vi "Init GUIs.vi"(0 "Windows in":T1, 1 "JSON":refnum<class "ConfigJSON.lvclass">, 2 "SVW":refnum<class "SharedVariableWrapper.lvclass">, 11 "error in":errorcluster) -> (4 "Windows out":T1, 15 "error out":errorcluster)   [LabVIEW 2019]
uses:
  TypeDef/Windows.ctl
  GUI Sensor Lib/GUI Sensor Lib.lvclass
  D:/GIT H4000/H4000/src/GUI_class/GUI.lvclass
  GUI Alarm Setting/GUI Alarm Setting.lvclass
  GUI Data Viewer_class/GUI Data Viewer.lvclass
  GUI Test Channels_class/GUI Test Channels.lvclass
  GUI Setting_class/GUI Setting.lvclass
  GUI Test HIPRESS_class/GUI Test HIPRESS.lvclass
  GUI NV class/GUI NV.lvclass
  GUI Work Windows_class/GUI Work Windows.lvclass
  PumpMotorGroup_class/GUI PumpMotorGroup.lvclass
  SV_Wrap/SharedVariableWrapper.lvclass
  ConfigJSON_class/ConfigJSON.lvclass
  D:/GIT H4000/H4000/src/ConfigInterface_class/ConfigInterface.lvclass
  GUI_class/GUI.lvclass/GUI.ctl
  GUI_class/GUI.lvclass
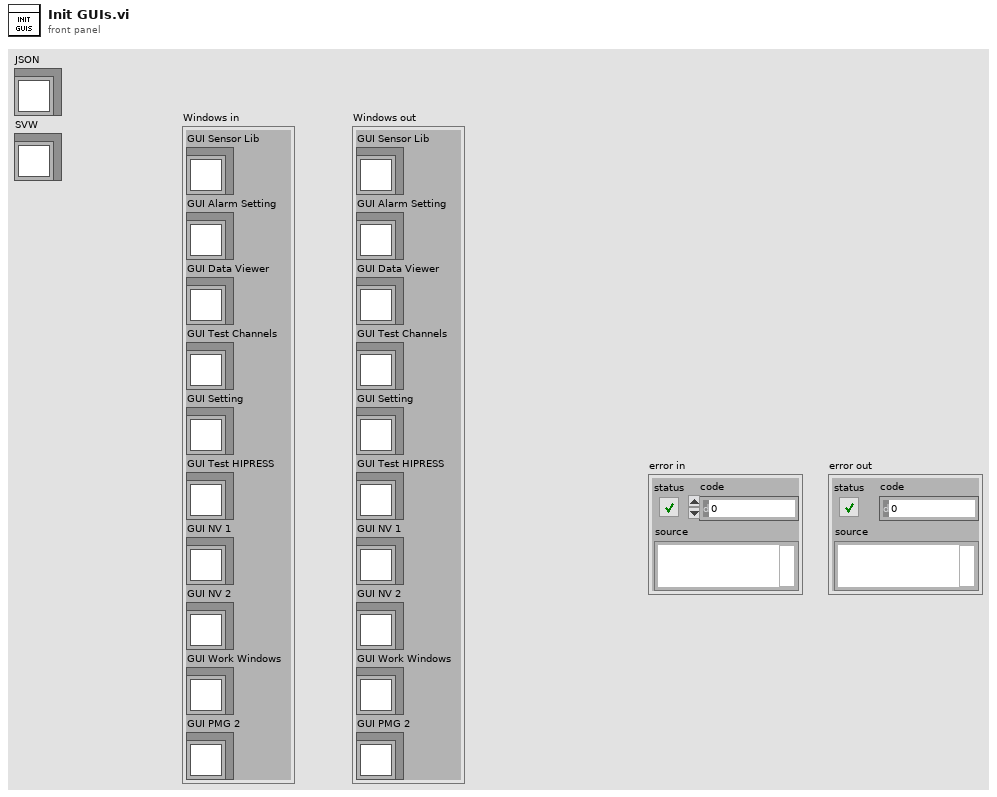
[diagram p1: front panel]
types:
  T1 = typedef "Windows.ctl" = cluster{"GUI Sensor Lib":refnum<class "GUI Sensor Lib.lvclass">, "GUI Alarm Setting":refnum<class "GUI Alarm Setting.lvclass">, "GUI Data Viewer":refnum<class "GUI Data Viewer.lvclass">, "GUI Test Channels":refnum<class "GUI Test Channels.lvclass">, "GUI Setting":refnum<class "GUI Setting.lvclass">, "GUI Test HIPRESS":refnum<class "GUI Test HIPRESS.lvclass">, "GUI NV 1":refnum<class "GUI NV.lvclass">, "GUI NV 2":refnum<class "GUI NV.lvclass">, "GUI Work Windows":refnum<class "GUI Work Windows.lvclass">, "GUI PMG 2":refnum<class "GUI PumpMotorGroup.lvclass">}
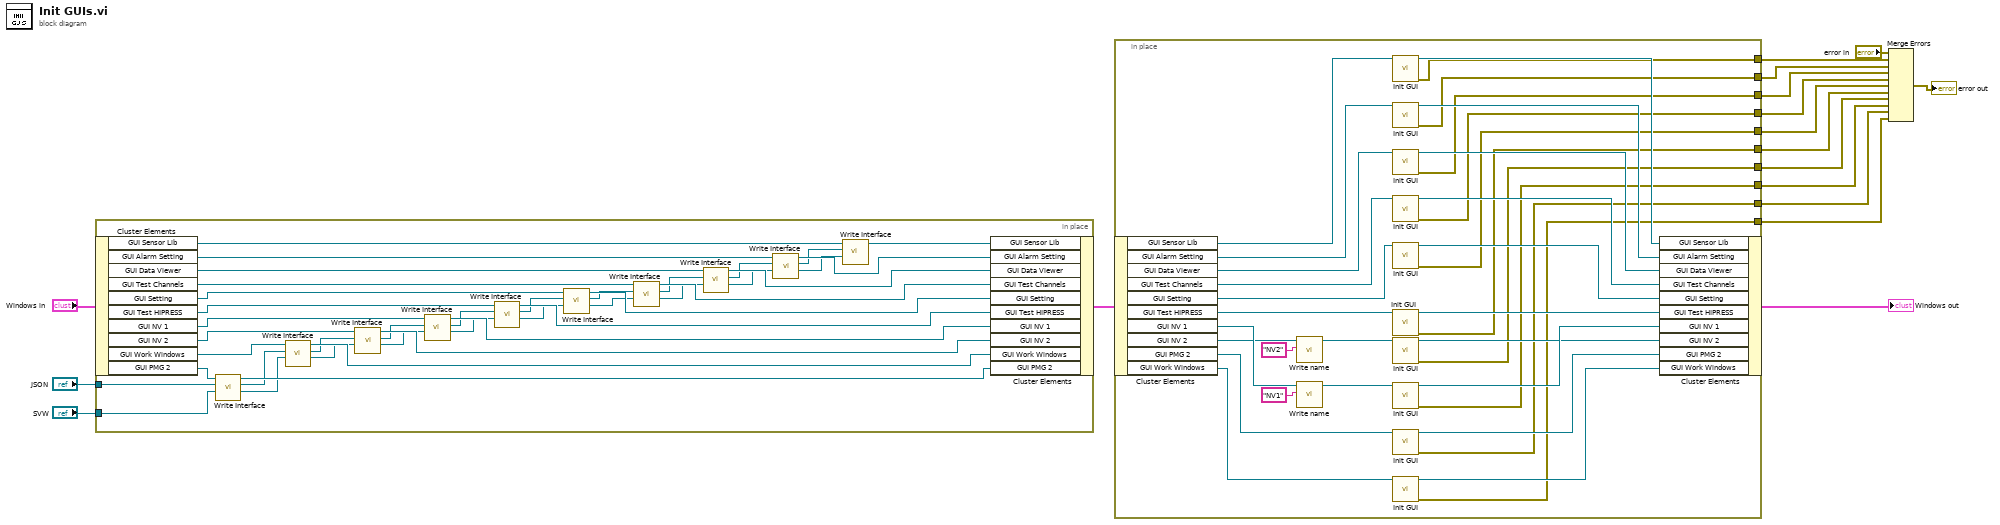
[diagram p0: block diagram]
diagram:
  n1 = in-place {
    in-place-border: "JSON" -> [w37]
    in-place-border: "SVW" -> [w36]
    n2 = in-place-cluster #1("Windows in") -> ("GUI Sensor Lib"=w57:refnum<class "GUI Sensor Lib.lvclass">, "GUI Alarm Setting"=w55:refnum<class "GUI Alarm Setting.lvclass">, "GUI Data Viewer"=w54:refnum<class "GUI Data Viewer.lvclass">, "GUI Test Channels"=w53:refnum<class "GUI Test Channels.lvclass">, "GUI Setting"=w52:refnum<class "GUI Setting.lvclass">, "GUI Test HIPRESS"=w51:refnum<class "GUI Test HIPRESS.lvclass">, "GUI NV 1"=w50:refnum<class "GUI NV.lvclass">, "GUI NV 2"=w49:refnum<class "GUI NV.lvclass">, "GUI Work Windows"=w48:refnum<class "GUI Work Windows.lvclass">, "GUI PMG 2"=w47:refnum<class "GUI PumpMotorGroup.lvclass">)
    n3 = call "Write Interface.vi"("SVW"=w36, "ConfigInterface"=w37, "GUI in"=w47) -> ("SVW 2"=w34:refnum<class "SharedVariableWrapper.lvclass">, "ConfigInterface 2"=w35:refnum<class "ConfigJSON.lvclass">, "GUI out"=w46:refnum<class "GUI PumpMotorGroup.lvclass">)  [unwired: 6 in]
    n4 = call "Write Interface.vi"("SVW"=w34, "ConfigInterface"=w35, "GUI in"=w48) -> ("SVW 2"=w25:refnum<class "SharedVariableWrapper.lvclass">, "ConfigInterface 2"=w33:refnum<class "ConfigJSON.lvclass">, "GUI out"=w45:refnum<class "GUI Work Windows.lvclass">)  [unwired: 6 in]
    n5 = call "Write Interface.vi"("SVW"=w25, "ConfigInterface"=w33, "GUI in"=w49) -> ("SVW 2"=w24:refnum<class "SharedVariableWrapper.lvclass">, "ConfigInterface 2"=w32:refnum<class "ConfigJSON.lvclass">, "GUI out"=w44:refnum<class "GUI NV.lvclass">)  [unwired: 6 in]
    n6 = call "Write Interface.vi"("SVW"=w24, "ConfigInterface"=w32, "GUI in"=w50) -> ("SVW 2"=w23:refnum<class "SharedVariableWrapper.lvclass">, "ConfigInterface 2"=w31:refnum<class "ConfigJSON.lvclass">, "GUI out"=w43:refnum<class "GUI NV.lvclass">)  [unwired: 6 in]
    n7 = call "Write Interface.vi"("SVW"=w23, "ConfigInterface"=w31, "GUI in"=w51) -> ("SVW 2"=w22:refnum<class "SharedVariableWrapper.lvclass">, "ConfigInterface 2"=w30:refnum<class "ConfigJSON.lvclass">, "GUI out"=w42:refnum<class "GUI Test HIPRESS.lvclass">)  [unwired: 6 in]
    n8 = call "Write Interface.vi"("SVW"=w22, "ConfigInterface"=w30, "GUI in"=w52) -> ("SVW 2"=w21:refnum<class "SharedVariableWrapper.lvclass">, "ConfigInterface 2"=w29:refnum<class "ConfigJSON.lvclass">, "GUI out"=w41:refnum<class "GUI Setting.lvclass">)  [unwired: 6 in]
    n9 = call "Write Interface.vi"("SVW"=w21, "ConfigInterface"=w29, "GUI in"=w53) -> ("SVW 2"=w20:refnum<class "SharedVariableWrapper.lvclass">, "ConfigInterface 2"=w28:refnum<class "ConfigJSON.lvclass">, "GUI out"=w40:refnum<class "GUI Test Channels.lvclass">)  [unwired: 6 in]
    n10 = call "Write Interface.vi"("SVW"=w20, "ConfigInterface"=w28, "GUI in"=w54) -> ("SVW 2"=w19:refnum<class "SharedVariableWrapper.lvclass">, "ConfigInterface 2"=w27:refnum<class "ConfigJSON.lvclass">, "GUI out"=w39:refnum<class "GUI Data Viewer.lvclass">)  [unwired: 6 in]
    n11 = call "Write Interface.vi"("SVW"=w19, "ConfigInterface"=w27, "GUI in"=w55) -> ("SVW 2"=w18:refnum<class "SharedVariableWrapper.lvclass">, "ConfigInterface 2"=w26:refnum<class "ConfigJSON.lvclass">, "GUI out"=w38:refnum<class "GUI Alarm Setting.lvclass">)  [unwired: 6 in]
    n12 = call "Write Interface.vi"("SVW"=w18, "ConfigInterface"=w26, "GUI in"=w57) -> ("GUI out"=w56:refnum<class "GUI Sensor Lib.lvclass">)  [unwired: 6 in, 2 out]
    n13 = in-place-cluster #1("GUI Sensor Lib"=w56, "GUI Alarm Setting"=w38, "GUI Data Viewer"=w39, "GUI Test Channels"=w40, "GUI Setting"=w41, "GUI Test HIPRESS"=w42, "GUI NV 1"=w43, "GUI NV 2"=w44, "GUI Work Windows"=w45, "GUI PMG 2"=w46) -> (w13:T1)
  }
  n14 = in-place {
    in-place-border: [w67] -> w12
    in-place-border: [w66] -> w11
    in-place-border: [w65] -> w10
    in-place-border: [w64] -> w9
    in-place-border: [w63] -> w8
    in-place-border: [w62] -> w7
    in-place-border: [w61] -> w6
    in-place-border: [w60] -> w5
    in-place-border: [w59] -> w4
    in-place-border: [w58] -> w3
    n15 = in-place-cluster #2(w13) -> ("GUI Sensor Lib"=w91:refnum<class "GUI Sensor Lib.lvclass">, "GUI Alarm Setting"=w89:refnum<class "GUI Alarm Setting.lvclass">, "GUI Data Viewer"=w87:refnum<class "GUI Data Viewer.lvclass">, "GUI Test Channels"=w85:refnum<class "GUI Test Channels.lvclass">, "GUI Setting"=w83:refnum<class "GUI Setting.lvclass">, "GUI Test HIPRESS"=w81:refnum<class "GUI Test HIPRESS.lvclass">, "GUI NV 1"=w78:refnum<class "GUI NV.lvclass">, "GUI NV 2"=w74:refnum<class "GUI NV.lvclass">, "GUI PMG 2"=w71:refnum<class "GUI PumpMotorGroup.lvclass">, "GUI Work Windows"=w69:refnum<class "GUI Work Windows.lvclass">)
    n16 = call "Write name.vi"("name"="NV2", "GUI in"=w74) -> ("GUI out"=w73:refnum<class "GUI NV.lvclass">)  [unwired: 9 in]
    n17 = call "Write name.vi"("name"="NV1", "GUI in"=w78) -> ("GUI out"=w76:refnum<class "GUI NV.lvclass">)  [unwired: 9 in]
    n18 = call-dynamic "Init GUI.vi"("GUI in"=w91) -> ("GUI"=w90:refnum<class "GUI Sensor Lib.lvclass">, "error out"=w58:errorcluster)  [unwired: 13 in]
    n19 = call-dynamic "Init GUI.vi"("GUI in"=w89) -> ("GUI"=w88:refnum<class "GUI Alarm Setting.lvclass">, "error out"=w59:errorcluster)  [unwired: 13 in]
    n20 = call-dynamic "Init GUI.vi"("GUI in"=w87) -> ("GUI"=w86:refnum<class "GUI Data Viewer.lvclass">, "error out"=w60:errorcluster)  [unwired: 13 in]
    n21 = call-dynamic "Init GUI.vi"("GUI in"=w85) -> ("GUI"=w84:refnum<class "GUI Test Channels.lvclass">, "error out"=w61:errorcluster)  [unwired: 13 in]
    n22 = call-dynamic "Init GUI.vi"("GUI in"=w83) -> ("GUI"=w82:refnum<class "GUI Setting.lvclass">, "error out"=w62:errorcluster)  [unwired: 13 in]
    n23 = call-dynamic "Init GUI.vi"("GUI in"=w81) -> ("GUI"=w80:refnum<class "GUI Test HIPRESS.lvclass">, "error out"=w63:errorcluster)  [unwired: 13 in]
    n24 = call-dynamic "Init GUI.vi"("GUI in"=w73) -> ("GUI"=w72:refnum<class "GUI NV.lvclass">, "error out"=w64:errorcluster)  [unwired: 13 in]
    n25 = call-dynamic "Init GUI.vi"("GUI in"=w76) -> ("GUI"=w79:refnum<class "GUI NV.lvclass">, "error out"=w65:errorcluster)  [unwired: 13 in]
    n26 = call-dynamic "Init GUI.vi"("GUI in"=w71) -> ("GUI"=w70:refnum<class "GUI PumpMotorGroup.lvclass">, "error out"=w66:errorcluster)  [unwired: 13 in]
    n27 = call-dynamic "Init GUI.vi"("GUI in"=w69) -> ("GUI"=w68:refnum<class "GUI Work Windows.lvclass">, "error out"=w67:errorcluster)  [unwired: 13 in]
    n28 = in-place-cluster #2("GUI Sensor Lib"=w90, "GUI Alarm Setting"=w88, "GUI Data Viewer"=w86, "GUI Test Channels"=w84, "GUI Setting"=w82, "GUI Test HIPRESS"=w80, "GUI NV 1"=w79, "GUI NV 2"=w72, "GUI PMG 2"=w70, "GUI Work Windows"=w68) -> (→"Windows out":T1)
  }
  n29 = Merge Errors("error in", w3, w4, w5, w6, w7, w8, w9, w10, w11, w12) -> (→"error out":errorcluster)
